vi "Fetch (Statistical).vi"(0 "VISA resource name":refnum<visa-resource-name>, 1 "Statistical Operation (0: Mean)":u16(ring) items=["Mean", "Standard Deviation", "Maximum", "Minimum", "Peak to Peak"], 5 "Timeout (10000 ms)":i32=10000 format="%#.6g", 11 "error in (no error)":errorcluster) -> (4 "VISA resource name out":refnum<visa-resource-name>, 6 "Statistical Operation Results":dbl[](array[numeric]), 15 "error out":errorcluster)   [LabVIEW 2018, in "Keithley 24XX.lvlib"]
doc: "Performs a calculation on the data in the trace buffer and fetches the result.\n\nThe data is returned in array form. If measurement data was used as the trace source, the array will hold a result for voltage, current, and resistance in that order. If not, the array will have a single element for the math or limit test calculation.\n\n<B>Note</B> Use this VI only with other low-level VIs. The high-level VIs automatically incorporate this functionality. This VI does not check the instrument status. If you want to check the instrument status, call the Error Query VI at the conclusion of the sequence."
uses:
  Keithley 24XX.lvlib
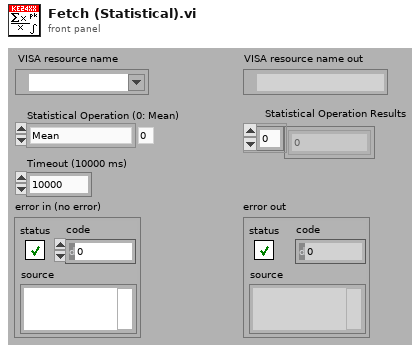
[diagram p1: front panel]
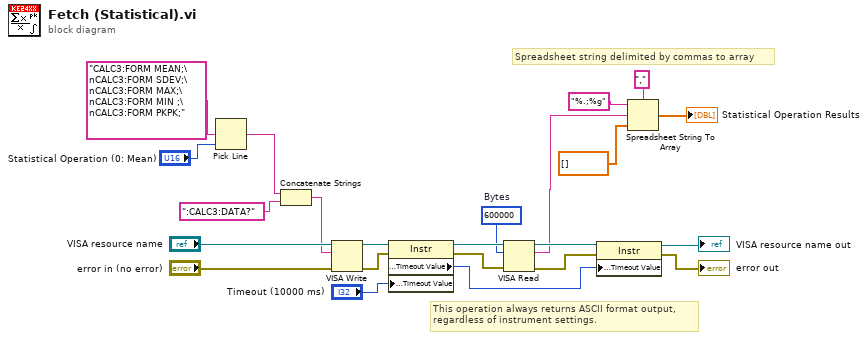
[diagram p0: block diagram]
diagram:
  w11 = u32 600000  # Bytes
  # "Spreadsheet string delimited by commas to array"
  # "This operation always returns ASCII format output, regardless of instrument settings."
  n1 = Pick Line(multi-line string="CALC3:FORM MEAN;\nCALC3:FORM SDEV;\nCALC3:FORM MAX;\nCALC3:FORM MIN ;\nCALC3:FORM PKPK;", line index="Statistical Operation (0: Mean)") -> (output string=w8:string)  [unwired: 1 in]
  n2 = Concatenate Strings(w8, ":CALC3:DATA?" ("string")) -> (w9:string)
  n3 = VISA Write(VISA resource name="VISA resource name", write buffer=w9, error in (no error)="error in (no error)") -> (VISA resource name out=w21:refnum<visa-resource-name>, error out=w20:errorcluster)  [unwired: 1 out]
  n4 = property class="Instr"(reference=w21, error in=w20, "General Settings:Timeout Value"="Timeout (10000 ms)") -> (reference out=w19:refnum<visa-resource-name>, error out=w18:errorcluster, "General Settings:Timeout Value"=w14:u32)
  n5 = VISA Read(VISA resource name=w19, byte count=w11, error in (no error)=w18) -> (VISA resource name out=w16:refnum<visa-resource-name>, read buffer=w5:string, error out=w15:errorcluster)  [unwired: 1 out]
  n6 = property class="Instr"(reference=w16, error in=w15, "General Settings:Timeout Value"=w14) -> (reference out=→"VISA resource name out":refnum<visa-resource-name>, error out=→"error out":errorcluster)
  n7 = Spreadsheet String To Array(delimiter (Tab)=",", format string="%.;%g", spreadsheet string=w5, array type (2D Dbl)=dbl[] []) -> (array=→"Statistical Operation Results":dbl[])
